vi "Read QD Raw Data.vi"(8 "Error In":errorcluster, 11 "KIT-QA in":refnum<class "KIT-QA.lvclass">) -> (0 "Error Out":errorcluster, 3 "KIT-QA out":refnum<class "KIT-QA.lvclass">)   [LabVIEW 2015, in "KIT-QA.lvlib" / "KIT-QA.lvclass"]
doc: "Read raw data of all enabled channels."
uses:
  KIT-QA.lvclass
  <vilib>/ActorFramework/Actor/Actor.lvclass/Actor.ctl
  <vilib>/ActorFramework/Message Enqueuer/Message Enqueuer.lvclass/Message Enqueuer.ctl
  KIT-QA.lvclass/KIT-QA.ctl
  <vilib>/ActorFramework/Message Enqueuer/Init from Existing Queue.vi
  <vilib>/ActorFramework/Message Enqueuer/Enqueue.vi
  <vilib>/Analysis/polynomials.llb/1D Polynomial Evaluation (DBL).vi
  <vilib>/Waveform/DWDTOps.llb/DWDT Boolean Array to Digital.vi
  <vilib>/ActorFramework/Message Priority Queue/Priority Enqueue.vi
  <vilib>/ActorFramework/Message Enqueuer/Message Enqueuer.lvclass
  KIT-QA Messages/Read DSC-Traces Msg/Read DSC-Traces Msg.lvclass
  <vilib>/ActorFramework/Actor/Actor.lvclass
  <vilib>/Analysis/NI_AALPro.lvlib
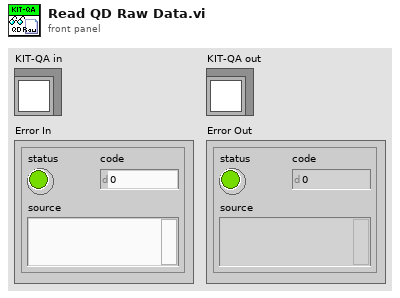
[diagram p1: front panel]
types:
  T1 = enum16{"open", "replace", "create", "open or create", "replace or create", "replace or create with confirmation"}
  T2 = cluster{"Calibration Factor":dbl[], "Unit":string}[]
  T3 = cluster{dbl[unit], i32, "digital waveform":digitalwaveform, waveform(dbl)[]}
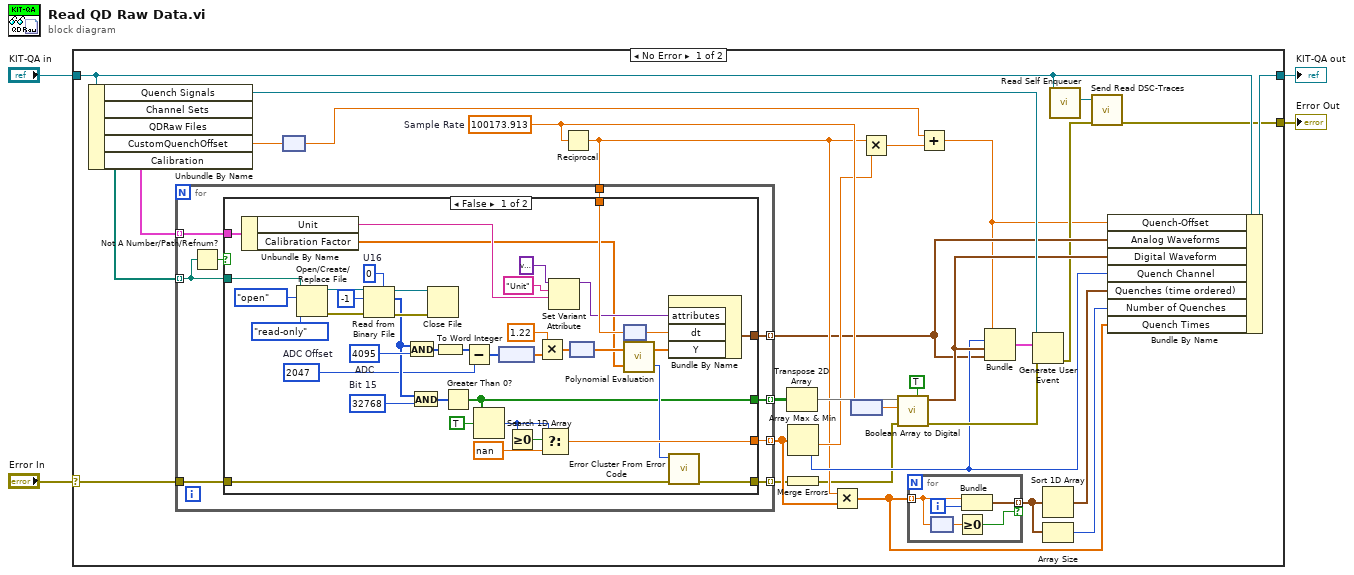
[diagram p0: block diagram]
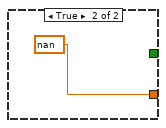
[diagram p2: hidden frame]
diagram:
  n1 = case shown="No Error" "Error In" {
    selector: "Error In" -> [w12 w93]
    tunnel: [w13 w93] -> w3
    tunnel: [w29 w92] -> w1
    tunnel: "KIT-QA in" -> [w16 w92]
    frame No Error {
      w33 = dbl[unit] 100173.913  # Sample Rate
      n2 = Unbundle By Name(w16) -> ("Quench Signals"=w27:refnum<user-event>, "QDRaw Files"=w30:path[], "CustomQuenchOffset"=w8:dbl, "Calibration"=w9:T2)  [unwired: 1 out]
      n3 = node(w8) -> (w5:dbl[unit])
      n4 = Reciprocal(x=w33) -> (1/x=w19:dbl[unit])
      n5 = for {
        tunnel: w30 -> [w46] mode=indexing
        tunnel: [w49] -> w18 mode=indexing
        tunnel: [w47] -> w24 mode=indexing
        tunnel: [w50] -> w36 mode=indexing
        tunnel: w19 -> [w48]
        tunnel: w9 -> [w44] mode=indexing
        tunnel: w12 -> [w43]
        tunnel: [w42] -> w11 mode=indexing
        n6 = Not A Number/Path/Refnum?(number/path/refnum=w46) -> (NaN/Path/Refnum?=w45:bool)
        n7 = case shown="False" w45 {
          tunnel: w46 -> [w81 _]
          tunnel: [w52 _] -> w50
          tunnel: [w76 _] -> w49
          tunnel: w48 -> [w72 _]
          tunnel: [w69 nan] -> w47
          tunnel: w44 -> [w58 _]
          tunnel: w43 -> [w53 _]
          tunnel: [w51 _] -> w42
          frame False {
            w66 = i16 2047  # ADC Offset
            w83 = u16 32768  # Bit 15
            w85 = u16 4095  # ADC
            w88 = u16 0  # U16
            n8 = Unbundle By Name(w58) -> ("Unit"=w56:string, "Calibration Factor"=w55:dbl[])
            n9 = Open/Create/Replace File(file path (use dialog)=w81, operation (0:open)=T1."open", access (0:read/write)=enum16{"read/write", "read-only", "write-only"}."read-only") -> (refnum out=w74:refnum<file>, error out=w73:errorcluster)  [unwired: 3 in, 1 out]
            n10 = Read from Binary File(5:w88, 8:w73, 10:-1 ("count (1)"), 11:w74) -> (0:w87:errorcluster, 2:w84:u16[], 3:w86:refnum<file>)  [unwired: 2 in, 1 out]
            n11 = And(x=w84, y=w85) -> (x .and. y?=w68:u16[])
            n12 = And(x=w84, y=w83) -> (x .and. y?=w82:u16[])
            n13 = Close File(refnum=w86, error in=w87) -> ()  [unwired: 2 out]
            n14 = To Word Integer(number=w68) -> (16bit integer=w65:i16[])
            n15 = Greater Than 0?(x=w82) -> (x > 0?=w52:bool[])
            n16 = Subtract(x=w65, y=w66) -> (x-y=w67:i16[])
            n17 = Search 1D Array(1D array=w52, element=TRUE) -> (index of element=w64:i32)  [unwired: 1 in]
            n18 = node(w67) -> (w79:dbl[unit][])
            n19 = Greater Or Equal To 0?(x=w64) -> (x >= 0?=w71:bool)
            n20 = Multiply(x=1.22 ("y"), y=w79) -> (x*y=w77:dbl[unit][])
            n21 = Select(t=w64, s=w71, f=nan) -> (s? t:f=w69:dbl)
            n22 = Set Variant Attribute(Variant=variant ("attributes"), name="Unit", value=w56) -> (Variant out=w61:variant)  [unwired: 1 in, 2 out]
            n23 = node(w77) -> (w59:dbl[])
            n24 = node(w72) -> (w63:dbl)
            n25 = call-poly <vilib>:"Polynomial Evaluation.vi"("P(x)"=w55, "A"=w59) -> ("error"=w54:i32, "P(A)"=w60:dbl[])
            n26 = Bundle By Name("attributes"=w61, "dt"=w63, "Y"=w60) -> (w76:waveform(dbl))  [unwired: 1 in]
            n27 = call <vilib>:"Error Cluster From Error Code.vi"("error in (no error)"=w53, "error code (0)"=w54) -> ("error out"=w51:errorcluster)  [unwired: 7 in]
          }
          frame True {
          }
        }
      }
      n28 = Transpose 2D Array(2D array=w36) -> (transposed array=w35:bool[][])
      n29 = Array Max & Min(array=w24) -> (min value=w32:dbl, min index (indices)=w21:i32)  [unwired: 2 out]
      n30 = Merge Errors(w11) -> (w10:errorcluster)
      n31 = Multiply(x=w19, y=w24) -> (x*y=w17:dbl[unit][])
      n32 = node(w33) -> (w31:dbl)
      n33 = Multiply(x=w19, y=w32) -> (x*y=w7:dbl[unit])
      n34 = call-poly <vilib>:"Boolean Array to Digital.vi"("compress data (F)"=TRUE, "error in (no error)"=w10, "sample rate"=w31, "boolean array"=w35) -> ("error out"=w28:errorcluster, "digital waveform"=w26:digitalwaveform)  [unwired: 6 in]
      n35 = for {
        tunnel: [w41] -> w25 mode=indexing if=w39
        tunnel: w17 -> [w38] mode=indexing
        i -> [w40]
        n36 = node(w38) -> (w37:dbl)
        n37 = Greater Or Equal To 0?(x=w37) -> (x >= 0?=w39:bool)
        n38 = Bundle(w38, w40) -> (w41:cluster{dbl[unit], i32})  [unwired: 1 in]
      }
      n39 = Add(x=w5, y=w7) -> (x+y=w6:dbl[unit])
      n40 = Bundle(w6, w21, "digital waveform"=w26, w18) -> (w20:T3)  [unwired: 1 in]
      n41 = Generate User Event(user event=w27, event data cluster=w20, error in=w28) -> (error out=w14:errorcluster)  [unwired: 1 in, 1 out]
      n42 = Sort 1D Array(array=w25) -> (sorted array=w23:cluster{dbl[unit], i32}[])
      n43 = Array Size(array=w25) -> (size(s)=w22:i32)
      n44 = call <vilib>:"Read Self Enqueuer.vi"("Actor"=w16) -> ("Self Enqueuer"=w15:refnum<class "Message Enqueuer.lvclass">)  [unwired: 10 in]
      n45 = call "Send Read DSC-Traces.vi"("error in (no error)"=w14, "Message Enqueuer"=w15) -> ("error out"=w13:errorcluster)  [unwired: 8 in, 1 out]
      n46 = Bundle By Name(cluster=w16, "Quench-Offset"=w6, "Analog Waveforms"=w18, "Digital Waveform"=w26, "Quench Channel"=w21, "Quenches (time ordered)"=w23, "Number of Quenches"=w22, "Quench Times"=w17) -> (w29:refnum<class "KIT-QA.lvclass">)
    }
    frame Error {
    }
  }
  "Error Out" <- w3
  "KIT-QA out" <- w1
